vi "findfltr.vi"(1 "Present Wavelength":dbl format="%.2f") -> (0 "Filter":i32=1 min=1 max=6 step=1)   [LabVIEW 2017]
doc: "Returns the grating position for the Present Wavelength parameter.\nUses the Globals \"Grat Wave Table\" and \"Grat Position Table\""
uses:
  m_globals.vi
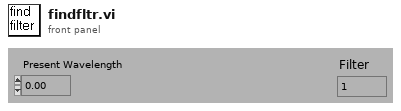
[diagram p1: front panel]
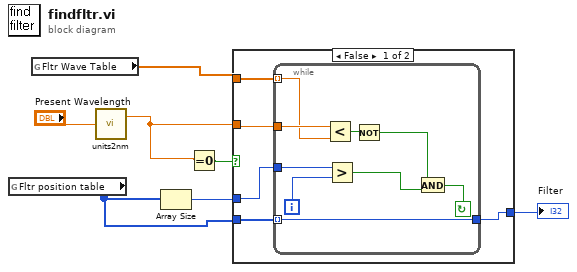
[diagram p0: block diagram]
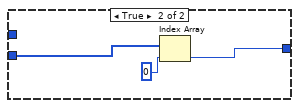
[diagram p2: hidden frame]
diagram:
  n1 = global read "m_globals.vi" "Fltr position table"() -> (w4:u16[])
  n2 = global read "m_globals.vi" "Fltr Wave Table"() -> (w1:dbl[])
  n3 = call "units2nm.vi"("Wavelength units"="Present Wavelength") -> ("Wavelength nm"=w2:dbl)  [unwired: 1 out]
  n4 = Array Size(array=w4) -> (size(s)=w5:i32)
  n5 = Equal To 0?(x=w2) -> (x = 0?=w3:bool)
  n6 = case shown="False" w3 {
    tunnel: w2 -> [w12 _]
    tunnel: w5 -> [w10 _]
    tunnel: w1 -> [w11 _]
    tunnel: w4 -> [w9 w22]
    tunnel: [w8 w23] -> w6
    frame False {
      n7 = while {
        tunnel: [w13] -> w8
        tunnel: w9 -> [w13] mode=indexing
        tunnel: w10 -> [w16]
        tunnel: w11 -> [w20] mode=indexing
        tunnel: w12 -> [w21]
        i -> [w15]
        stop <- w19 continue-if-true
        n8 = Less?(x=w21, y=w20) -> (x < y?=w18:bool)
        n9 = Greater?(x=w16, y=w15) -> (0:w14:bool)
        n10 = Not(x=w18) -> (.not. x?=w17:bool)
        n11 = And(x=w17, y=w14) -> (x .and. y?=w19:bool)
      }
    }
    frame True {
      n12 = Index Array(array=w22, index=0) -> (element=w23:u16)
    }
  }
  "Filter" <- w6
